vi "Read Event Source Enqueuer.vi"(8 "error in (no error)":errorcluster, 11 "Event Sink in":refnum<class "Event Sink.lvclass">) -> (0 "error out":errorcluster, 2 "Actor Framework:Message Enqueuer":refnum<class "Message Enqueuer.lvclass">, 3 "Event Sink out":refnum<class "Event Sink.lvclass">)   [LabVIEW 2016, in "Event Source.lvlib" / "Event Sink.lvclass"]
uses:
  Event Sink.lvclass
  <vilib>/ActorFramework/Message Enqueuer/Message Enqueuer.lvclass
  Event Sink.lvclass/Event Sink.ctl
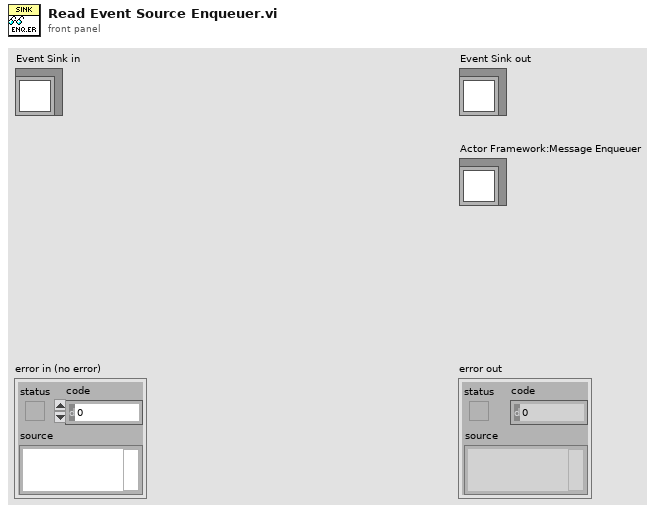
[diagram p1: front panel]
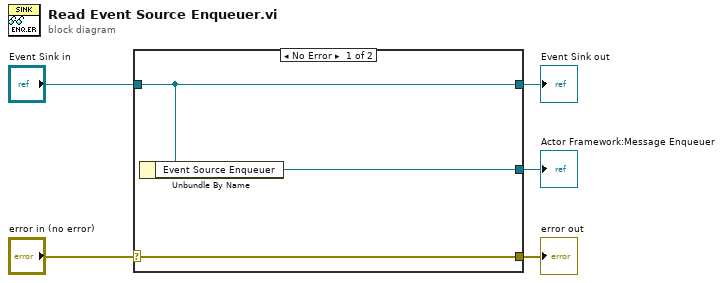
[diagram p0: block diagram]
diagram:
  n1 = case shown="No Error" "error in (no error)" {
    selector: "error in (no error)" -> [w8 w9]
    tunnel: [w8 w9] -> w4
    tunnel: [w7 w10] -> w2
    tunnel: "Event Sink in" -> [w7 w10]
    tunnel: [w6 _] -> w1
    frame No Error {
      n2 = Unbundle By Name(w7) -> ("Event Source Enqueuer"=w6:refnum<class "Message Enqueuer.lvclass">)
    }
    frame Error {
    }
  }
  "error out" <- w4
  "Event Sink out" <- w2
  "Actor Framework:Message Enqueuer" <- w1
